vi "Set Hardware Manager.vi"(8 "error in (no error)":errorcluster, 10 "HardwareManager":refnum<class "HardwareManager.lvclass">=refnum, 11 "Sequencer in":refnum<class "Sequencer.lvclass">=refnum) -> (0 "error out":errorcluster, 3 "Service out":refnum<class "Sequencer.lvclass">)   [LabVIEW 2020]
uses:
  Sequencer.lvclass
  HardwareManager/HardwareManager.lvclass
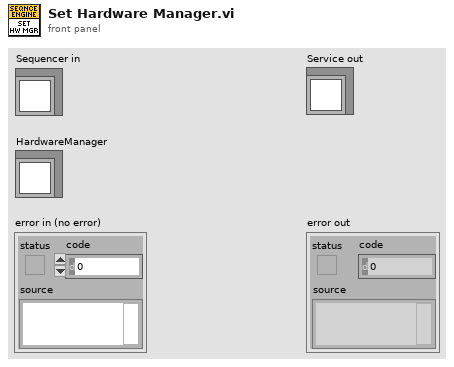
[diagram p1: front panel]
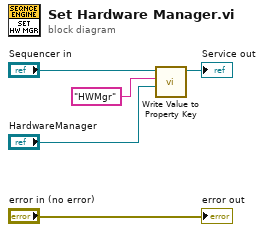
[diagram p0: block diagram]
diagram:
  n1 = call "Write Value to Property Key.vi"("Value"="HardwareManager", "Key"="HWMgr", "Service in"="Sequencer in") -> ("Service out"=→"Service out":refnum<class "Sequencer.lvclass">)  [unwired: 7 in, 1 out]
  "error out" <- "error in (no error)"
